vi "SA40144D.20210825 1D+2D.vi"() -> ()   [LabVIEW 2020]
uses:
  <userlib>/LevyLab/XY Utilities/subVIs/Linear Fit (single).vi
  <userlib>/LevyLab/LV to ITX/Data/Data.lvclass
  <userlib>/LevyLab/XY Utilities/xy_utilities.lvlib
panel:
  in  "Tab Control":enum32{"Page 1", "Page 2"}(tab)
  out "G4T vs t  2D":T1(graph)
  out "Temp vs time":T1(graph)
  out "G4T vs t":T1(graph)
  out "G2T vs t":T1(graph)
  out "Arrhenius":cluster{dbl[], dbl[]}[](graph)
  out "E_a":dbl[](array[numeric])
  in  "Source Voltage":dbl=0.1
  in  "Data Folder":path=path "G:/My Drive/ansom/Data/PPMS 2/SA40144D.20210825/45-LockinFieldSweep_hash_16_27_stripe/SA40144D.20210825.000000.dat"
  in  "Trimming":i32=400
  in  "Update":bool
  in  "OK":bool
  out "error out":errorcluster
  in  "error in (no error)":errorcluster
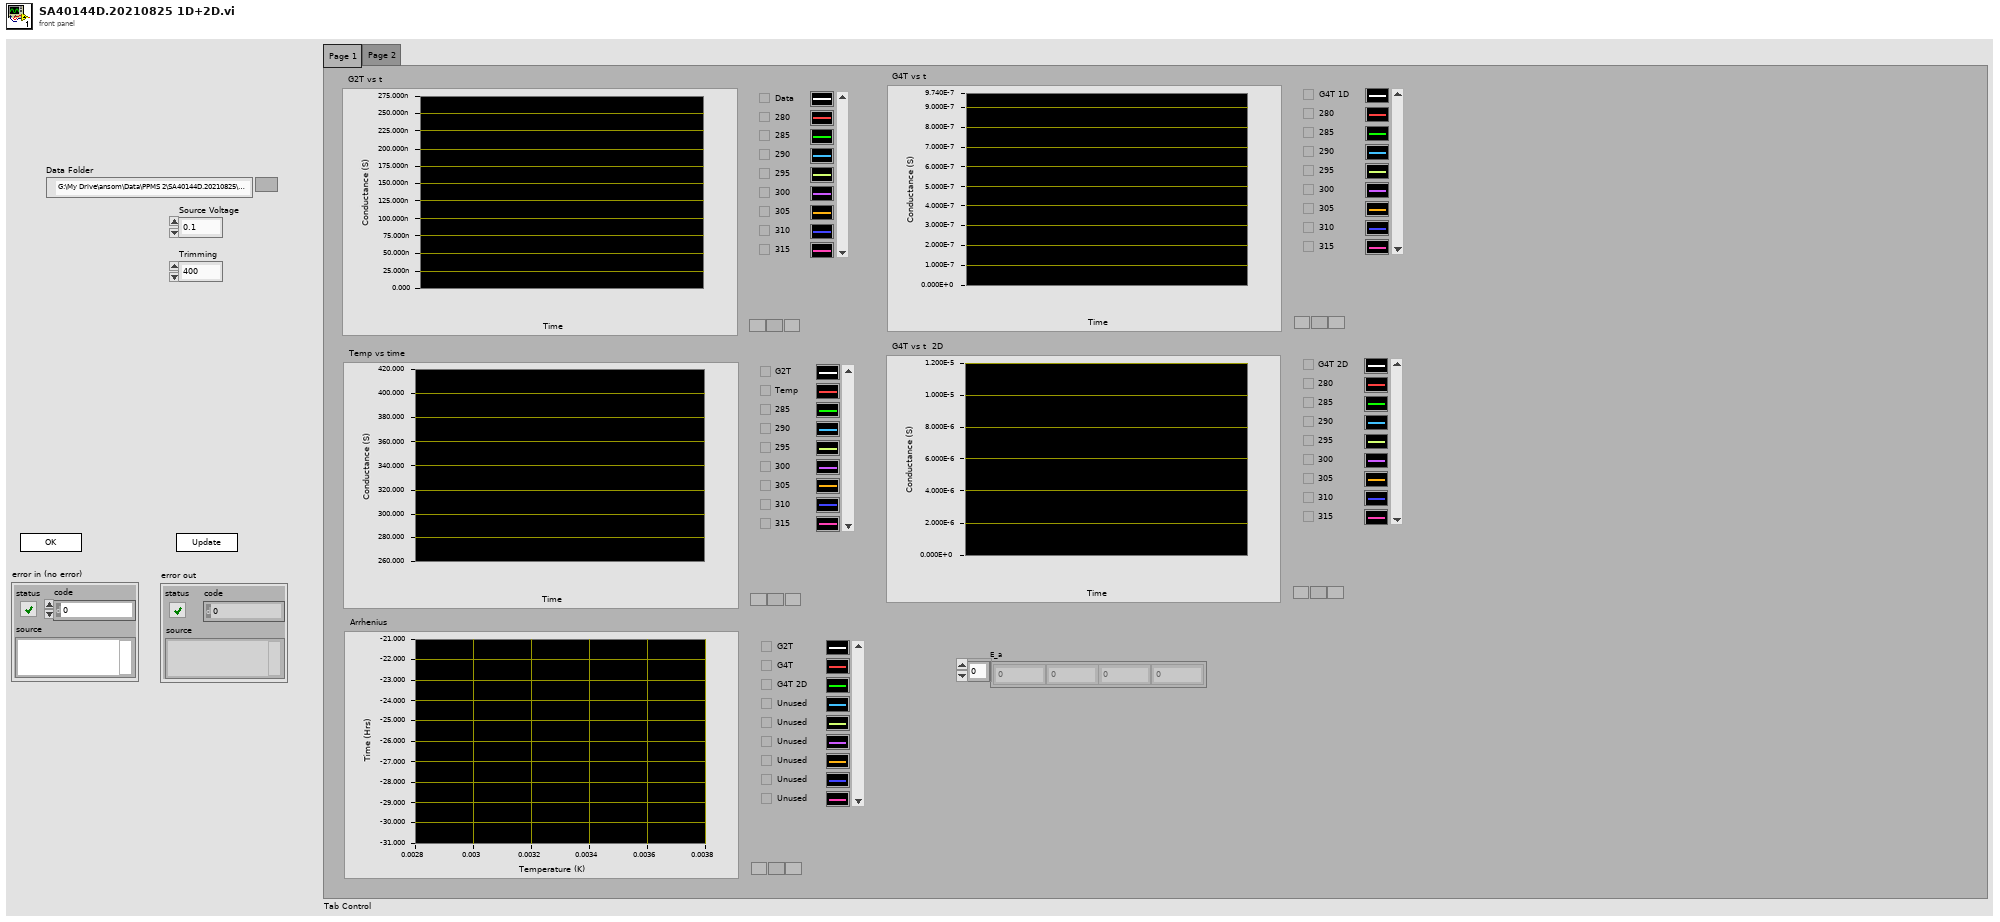
[diagram p1: front panel]
types:
  T1 = cluster{"Data":dbl[], "Best Exponential Fit":dbl[]}[]
  T2 = enum32{"Invalid", "Standard", "Closed", "Hidden", "Minimized", "Maximized"}
  T3 = enum32{"invalid app kind", "Development System", "Run Time System", "Student Edition", "Embedded LabVIEW", "Evaluation", "Custom"}
  T4 = cluster{"Core":cluster{"Current VI Reference":refnum<vi>, "Close Panel on Exit?":bool}, "G2T 1D":cluster{dbl[], dbl[]}[], "G4T 1D":cluster{dbl[], dbl[]}[], "G2T 2D":cluster{dbl[], dbl[]}[], "G4T 2D":cluster{dbl[], dbl[]}[], "Arrhenius":cluster{dbl[], dbl[]}[], "Source Voltage":dbl, "Data Folder":path, "Trimming":i32}
  T5 = cluster{"Current VI Reference":refnum<vi>, "Close Panel on Exit?":bool}
  T6 = typedef "Data.lvclass/Dictionary--cluster.ctl" = cluster{"key":string, "value":variant}
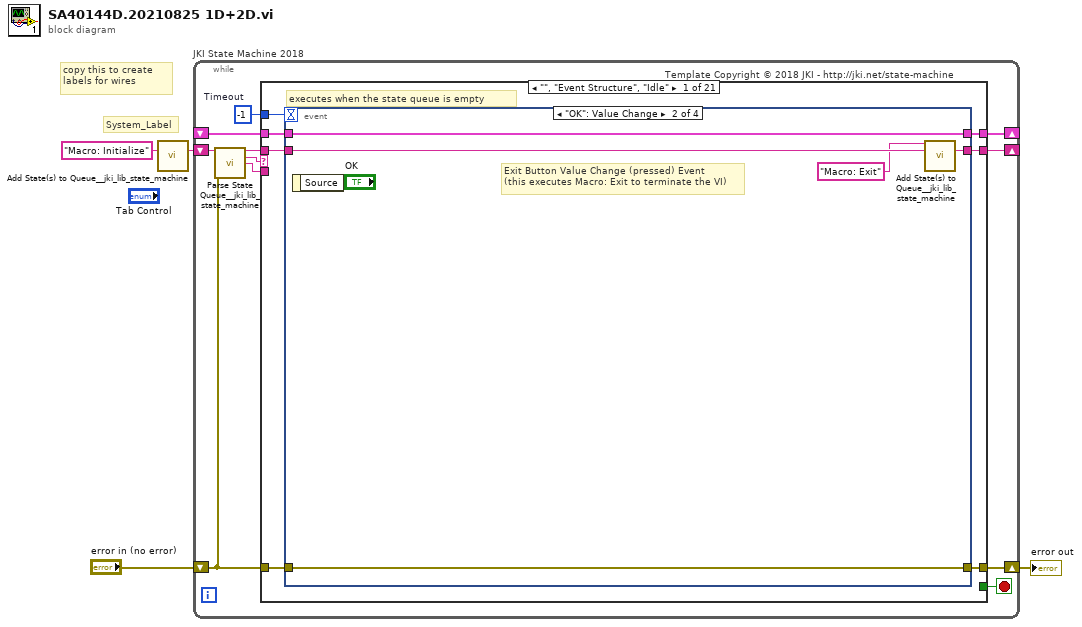
[diagram p0: block diagram]
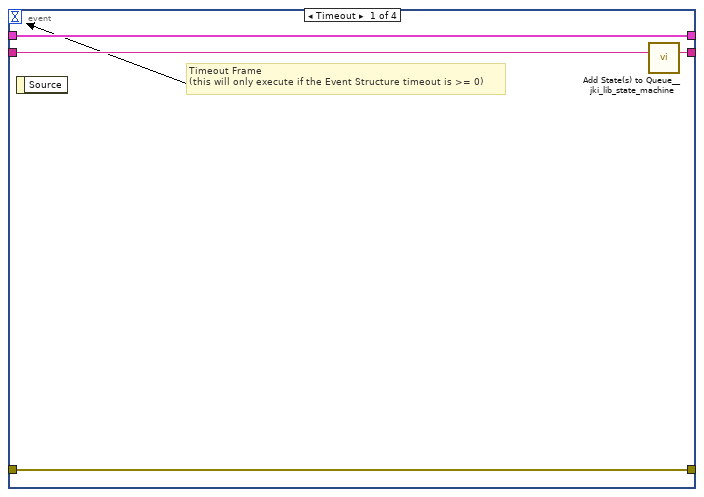
[diagram p2: hidden frame]
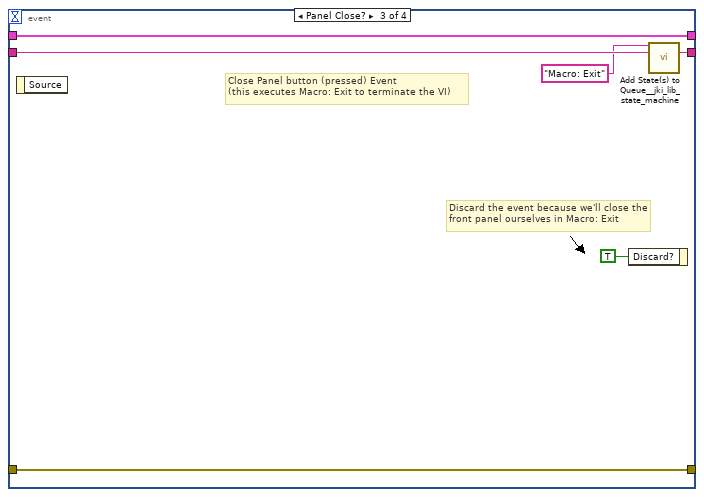
[diagram p3: hidden frame]
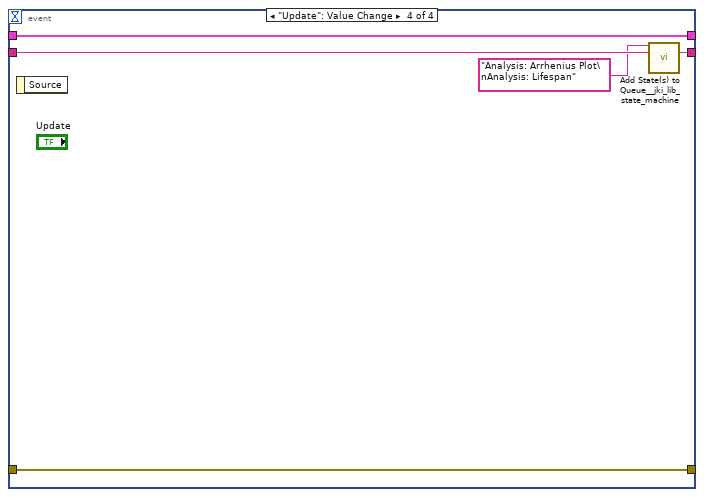
[diagram p4: hidden frame]
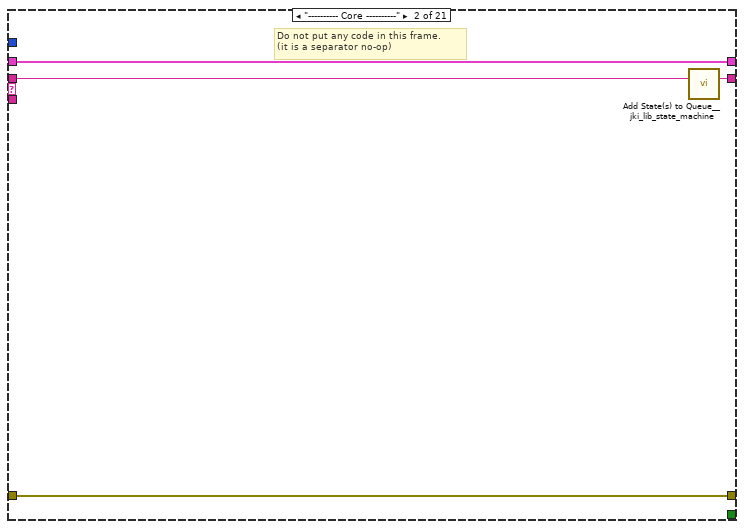
[diagram p5: hidden frame]
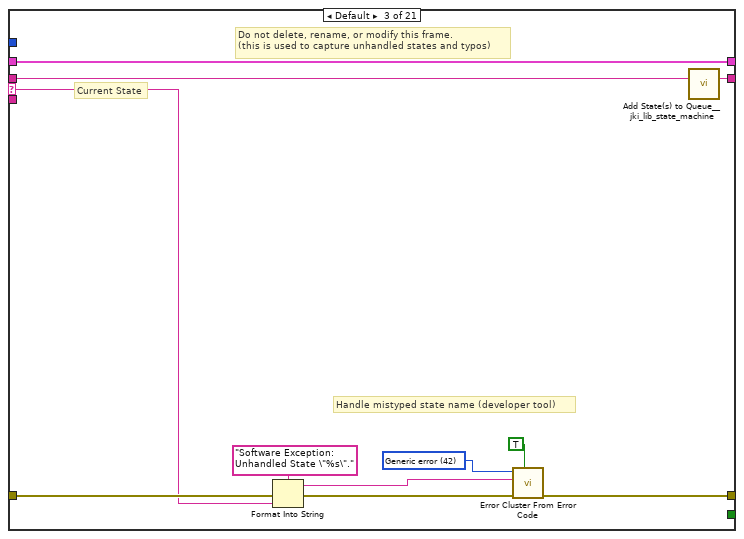
[diagram p6: hidden frame]
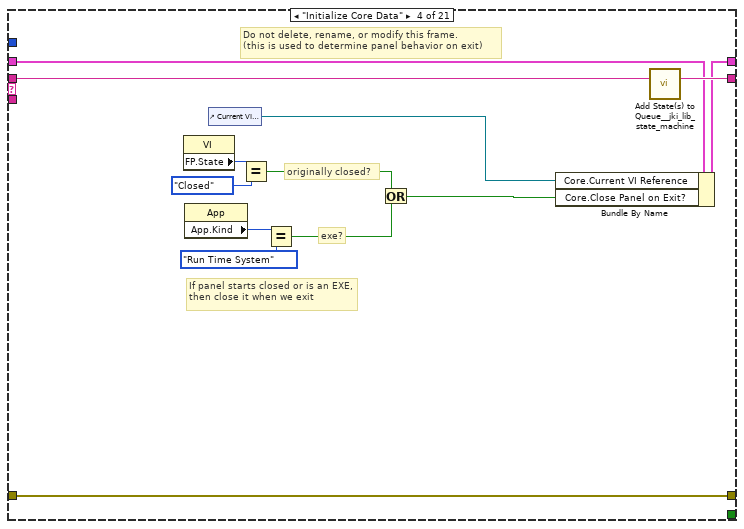
[diagram p7: hidden frame]
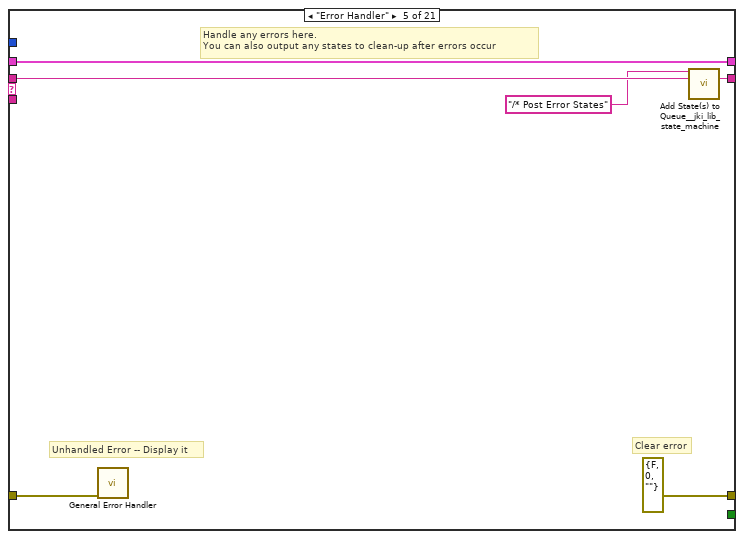
[diagram p8: hidden frame]
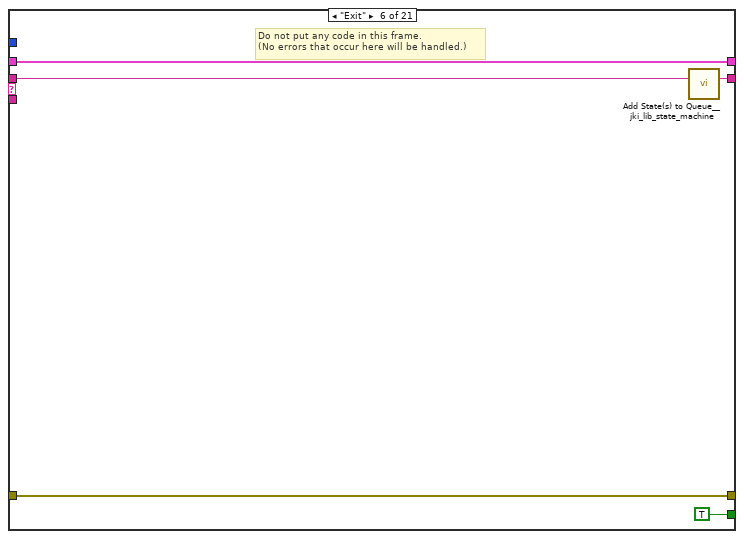
[diagram p9: hidden frame]
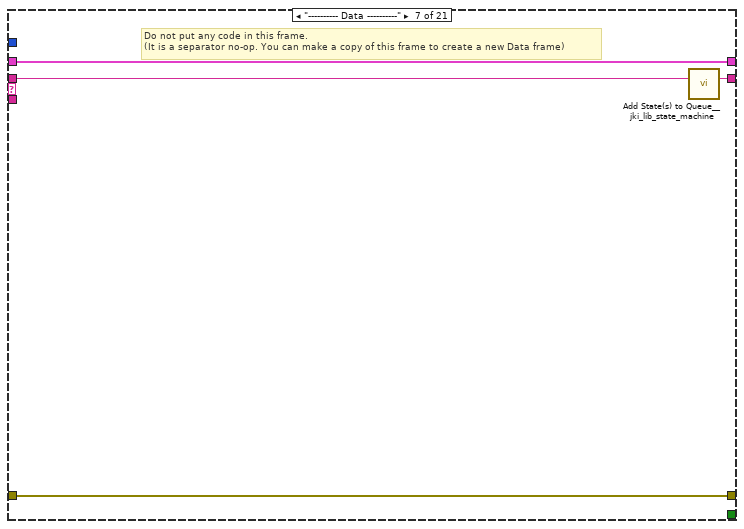
[diagram p10: hidden frame]
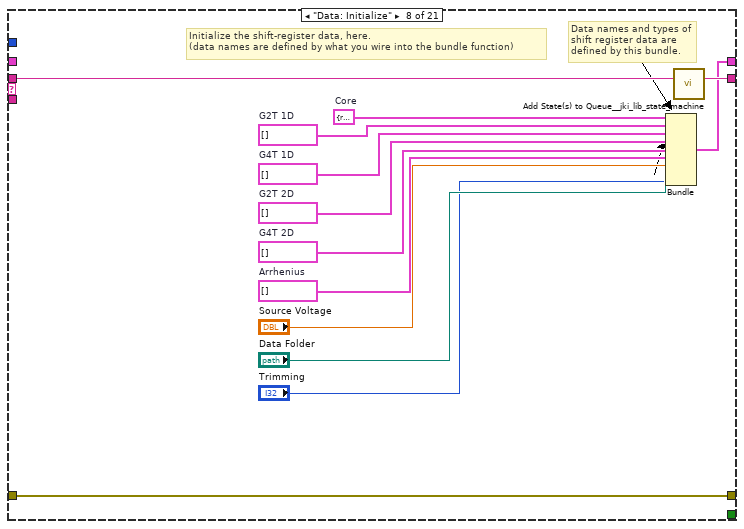
[diagram p11: hidden frame]
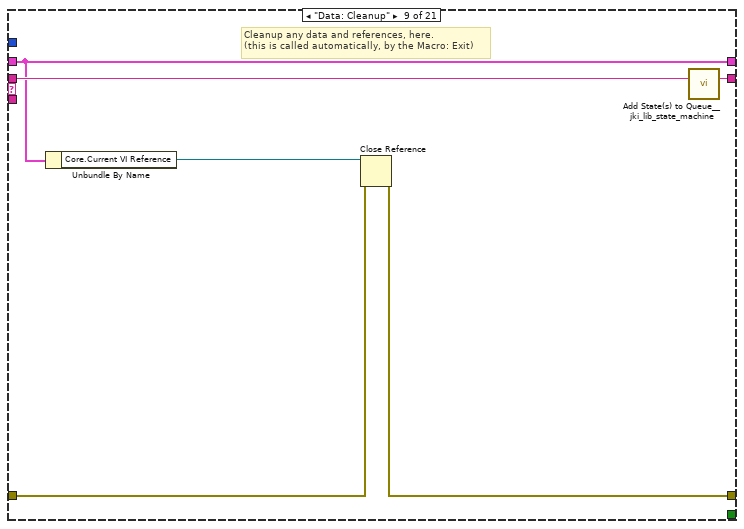
[diagram p12: hidden frame]
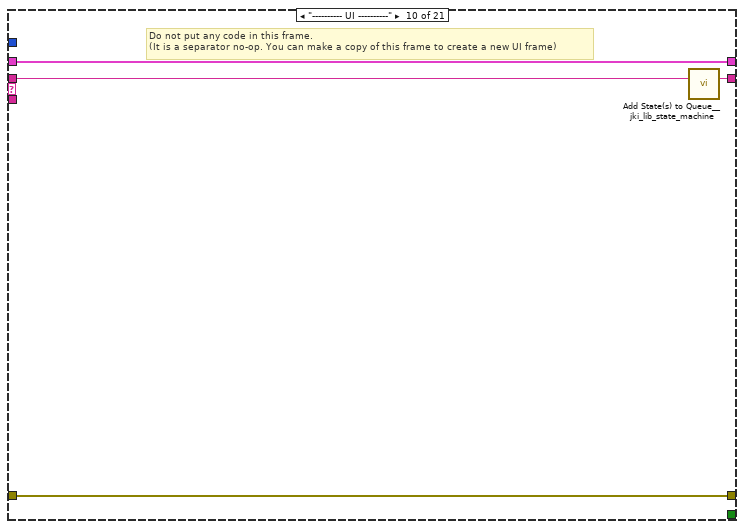
[diagram p13: hidden frame]
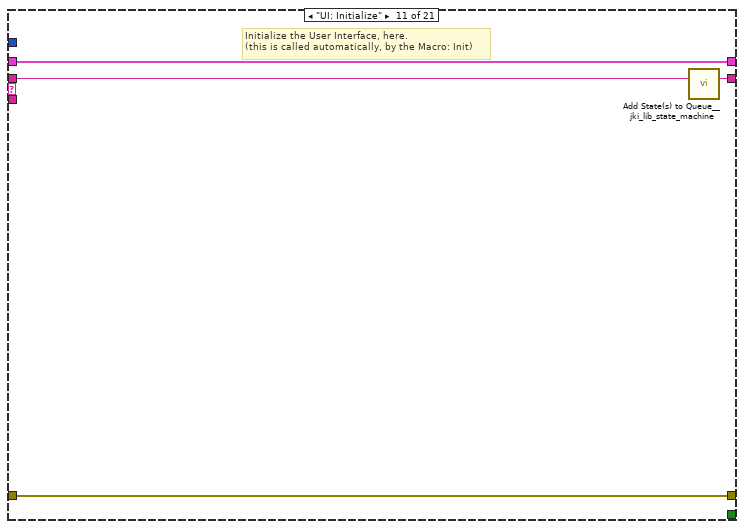
[diagram p14: hidden frame]
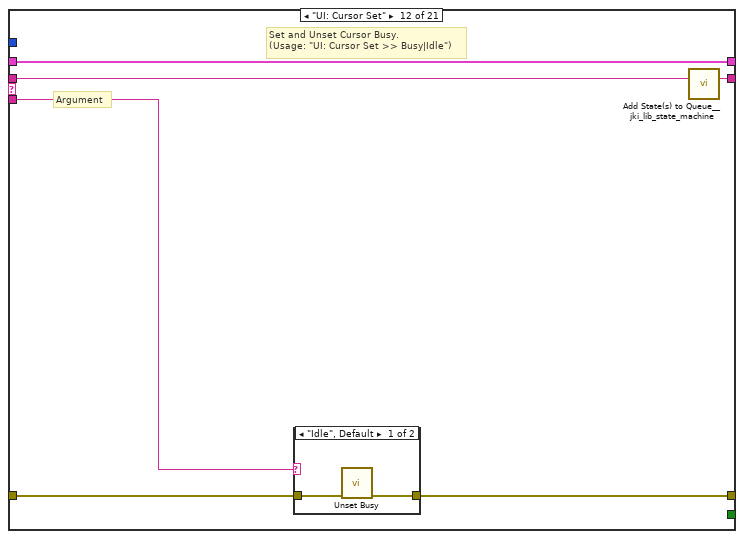
[diagram p15: hidden frame]
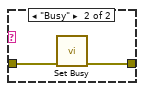
[diagram p16: hidden frame]
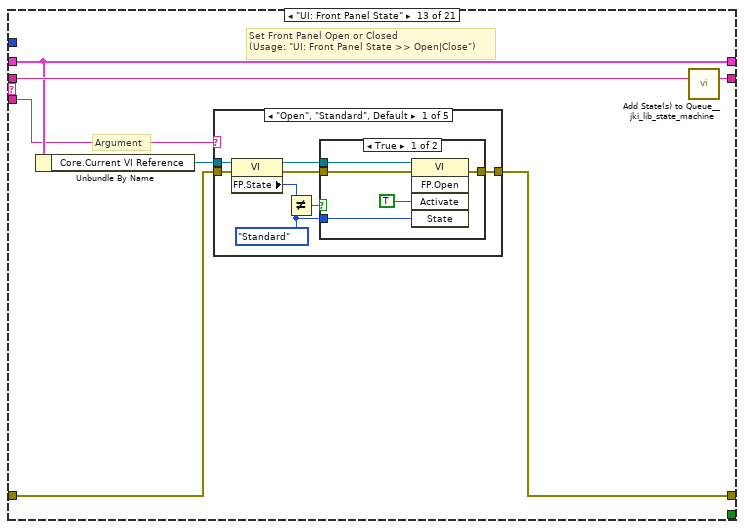
[diagram p17: hidden frame]
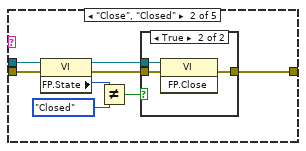
[diagram p19: hidden frame]
diagram:
  # "copy this to create labels for wires"
  # "System_Label"
  n1 = call <vilib>:"Add State(s) to Queue__jki_lib_state_machine.vi"("State(s) in (\"\")"="Macro: Initialize") -> ("States Out"=w4:string)  [unwired: 14 in]
  n2 = while "JKI State Machine 2018" {
    shift-right: [w8] -> _
    shift-left: _ -> [w7]
    shift-right: [w11] -> w1
    shift-left: "error in (no error)" -> [w5]
    shift-right: [w10] -> _
    shift-left: w4 -> [w12]
    stop <- w9 stop-if-true
    w6 = -1  # Timeout
    # "Template Copyright © 2018 JKI - http://jki.net/state-machine"
    n3 = call <vilib>:"Parse State Queue__jki_lib_state_machine.vi"("State Queue"=w12, "Error In (no error)"=w5) -> ("Remaining States"=w14:string, "Current State"=w15:string, "Arguments"=w13:string)  [unwired: 11 in]
    n4 = case shown="\"\", \"Event Structure\", \"Idle\"" w15 {
      selector: w15 -> [_ _ w47 _ _ _ _ _ _ _ _ _ _ _ _ _ _ _ _ _ _]
      tunnel: w14 -> [w22 w46 w51 w70 w76 w81 w85 w98 w104 w108 w112 w118 w129 w198 w203 w213 w217 w249 w280 w292 w311]
      tunnel: w13 -> [_ _ _ _ _ _ _ _ _ _ _ w113 w123 _ _ _ _ _ _ _ _]
      tunnel: w7 -> [w20 w43 w49 w63 w73 w79 w82 _ w99 w105 w110 w116 w125 w195 w200 w210 w214 w245 w276 w289 w296]
      tunnel: [w19 w44 w53 w67 errorcluster {"status"=FALSE, "code"=0, "source"=""} ("error out") w78 w83 w95 w100 w106 w109 w114 w126 w196 w201 w211 w215 w247 w278 w290 w309] -> w11
      tunnel: w5 -> [w18 w44 w52 w67 w72 w78 w83 w95 w101 w106 w109 w115 w127 w196 w201 w211 w215 w247 w278 w290 w309]
      tunnel: [w21 w45 w50 w69 w75 w80 w84 w97 w103 w107 w111 w117 w128 w197 w202 w212 w216 w248 w279 w291 w310] -> w10
      tunnel: [_ _ _ _ _ TRUE _ _ _ _ _ _ _ _ _ _ _ _ _ _ _] -> w9
      tunnel: [w17 w43 w49 w68 w73 w79 w82 w96 w99 w105 w110 w116 w125 w195 w200 w210 w214 w246 w277 w289 w297] -> w8
      tunnel: w6 -> [w16 _ _ _ _ _ _ _ _ _ _ _ _ _ _ _ _ _ _ _ _]
      frame "", "Event Structure", "Idle" {
        # "executes when the state queue is empty"
        n5 = event shown="[1] \"OK\": Value Change" {
          selector: _ -> [_ _ _ _]
          dyn-events: _ -> [_ _ _ _]
          timeout: w16 -> [_ _ _ _]
          tunnel: w22 -> [w26 w31 w37 w41]
          tunnel: [w25 w30 w36 w40] -> w21
          tunnel: w20 -> [w23 w28 w34 w42]
          tunnel: [w24 w29 w35 w38] -> w19
          tunnel: w18 -> [w24 w29 w35 w38]
          tunnel: [w23 w28 w34 w42] -> w17
          event Timeout {
            # "Timeout Frame\n(this will only execute if the Event Structure timeout is >= 0)"
            n6 = event-data() -> ()  [unwired: 1 in, 1 out]
            n7 = call <vilib>:"Add State(s) to Queue__jki_lib_state_machine.vi"("State(s) in (\"\")"=w26) -> ("States Out"=w25:string)  [unwired: 14 in]
          }
          event "OK": Value Change {
            # "Exit Button Value Change (pressed) Event\n(this executes Macro: Exit to terminate the VI)"
            n8 = event-data() -> ()  [unwired: 1 in, 1 out]
            n9 = call <vilib>:"Add State(s) to Queue__jki_lib_state_machine.vi"("State(s) in Front (\"\")"="Macro: Exit", "State(s) in (\"\")"=w31) -> ("States Out"=w30:string)  [unwired: 13 in]
          }
          event Panel Close? {
            # "Discard the event because we'll close the front panel ourselves in Macro: Exit"
            # "Close Panel button (pressed) Event\n(this executes Macro: Exit to terminate the VI)"
            n10 = event-data() -> ()  [unwired: 1 in, 1 out]
            n11 = event-data("Discard?"=TRUE) -> ()  [unwired: 1 in, 1 out]
            n12 = call <vilib>:"Add State(s) to Queue__jki_lib_state_machine.vi"("State(s) in Front (\"\")"="Macro: Exit", "State(s) in (\"\")"=w37) -> ("States Out"=w36:string)  [unwired: 13 in]
          }
          event "Update": Value Change {
            n13 = event-data() -> ()  [unwired: 1 in, 1 out]
            n14 = call <vilib>:"Add State(s) to Queue__jki_lib_state_machine.vi"("State(s) in Front (\"\")"="Analysis: Arrhenius Plot\nAnalysis: Lifespan" ("State(s) in Front (\"\")"), "State(s) in (\"\")"=w41) -> ("States Out"=w40:string)  [unwired: 13 in]
          }
        }
      }
      frame "---------- Core ----------" {
        # "Do not put any code in this frame.\n(it is a separator no-op)"
        n15 = call <vilib>:"Add State(s) to Queue__jki_lib_state_machine.vi"("State(s) in (\"\")"=w46) -> ("States Out"=w45:string)  [unwired: 14 in]
      }
      frame Default {
        w56 = 42 items=["No error", "Argument error", "Memory is full", "Out of zone", "End of file", "File already open", "Generic file I/O error", "File not found", "File permission error", "Disk is full", "Duplicate path", "Too many files open", "System feature not enabled", "Resource file not found", "Cannot add resource", "Resource not found", "Image not found", "Image memory error", "Pen does not exist", "Config type invalid", "Config token not found", "Config parse error", "Config memory error", "Bad external code format", "Bad external code offset", "External code not present", "Null window", "Destroy window error", "Null menu", "Print aborted", "Bad print record", "Print driver error", "Windows error during printing", "Memory error during printing", "Print dialog error", "Generic print error", "Invalid device refnum", "Device not found", "Device parameter error", "Device unit error", "Cannot open device", "Device call aborted", "Generic error", "Cancelled by user", "Object ID too low", "Object ID too high", "Object not in heap", "Unknown heap", "Unknown object (invalid DefProc)", "Unknown object (DefProc not in table)", "Message out of range", "Invalid (null) method", "Unknown message", "Manager call not supported", "Bad address", "Network operation in progress", "Network operation timed out", "Connection is busy", "Network attribute not supported", "Network error", "Address in use", "System out of memory", "Connection aborted", "Connection refused", "Not connected", "Already connected", "Connection closed", "Initialization error (interapplication manager)", "Bad occurrence", "Wait on unbound occurrence handler", "Occurrence queue overflow", "Datalog type conflict", "Unused", "Unrecognized type (interapplication manager)", "Memory corrupt", "Failed to make temporary DLL", "Old CIN version", "Drag socket not found", "Failed to load drop-object", "Failed to register OLE object", "Failed to release OLE object", "Format specifier type mismatch", "Unknown format specifier", "Too few format specifiers", "Too many format specifiers", "Scan failed", "Newer CIN version", "Error converting to variant", "Runtime menu error", "Password tampered", "Variant attribute not found", "Incompatible variant data type", "Event data is not available", "Event Store is not present", "Occurrence is not found", "Event Queue is not created", "Event info is not available", "Refnum passed is NULL", "Error retrieving Class GUID", "Error retrieving CoClass GUID", "Error retrieving TypeLib GUID.", "Bad built application magic bytes.", "Specific driver is different from the specific driver associated with the Logical Name.", "There is no session opened to the class driver.", "Max Error", "MAX - Error with config objects", "MAX - Error loading configuration", "MAX - Group not supported"]
        # "Current State"
        # "Do not delete, rename, or modify this frame.\n(this is used to capture unhandled states and typos)"
        # "Handle mistyped state name (developer tool)"
        n16 = Format Into String(format string="Software Exception: Unhandled State \"%s\"." ("message"), error in=w52, w47) -> (resulting string=w55:string, error out=w54:errorcluster)  [unwired: 1 in]
        n17 = call <vilib>:"Error Cluster From Error Code.vi"("show call chain? (False)"=TRUE, "error in (no error)"=w54, "error message (\"\")"=w55, "error code (0)"=w56) -> ("error out"=w53:errorcluster)  [unwired: 5 in]
        n18 = call <vilib>:"Add State(s) to Queue__jki_lib_state_machine.vi"("State(s) in (\"\")"=w51) -> ("States Out"=w50:string)  [unwired: 14 in]
      }
      frame "Initialize Core Data" {
        # "Do not delete, rename, or modify this frame.\n(this is used to determine panel behavior on exit)"
        # "originally closed?"
        # "exe?"
        # "If panel starts closed or is an EXE, then close it when we exit"
        n19 = property class="VI"() -> ("FP.State"=w60:T2)  [unwired: 2 in, 2 out]
        n20 = property class="App"() -> ("App.Kind"=w66:T3)  [unwired: 2 in, 2 out]
        n21 = control-ref of="Current VI Reference"() -> (w61:refnum<vi>)
        n22 = Equal?(x=w60, y=T2."Closed" ("Front Panel Window:State")) -> (x = y?=w58:bool)
        n23 = Equal?(x=w66, y=T3."Run Time System" ("Application:Kind")) -> (x = y?=w64:bool)
        n24 = Or(x=w58, y=w64) -> (x .or. y?=w62:bool)
        n25 = Bundle By Name(cluster=w63, "Core.Current VI Reference"=w61, "Core.Close Panel on Exit?"=w62) -> (w68:T4)
        n26 = call <vilib>:"Add State(s) to Queue__jki_lib_state_machine.vi"("State(s) in (\"\")"=w70) -> ("States Out"=w69:string)  [unwired: 14 in]
      }
      frame "Error Handler" {
        # "Unhandled Error -- Display it"
        # "Handle any errors here.\nYou can also output any states to clean-up after errors occur"
        # "Clear error"
        n27 = call <vilib>:"General Error Handler.vi"("error in (no error)"=w72) -> ()  [unwired: 10 in, 5 out]
        n28 = call <vilib>:"Add State(s) to Queue__jki_lib_state_machine.vi"("State(s) in Front (\"\")"="/* Post Error States", "State(s) in (\"\")"=w76) -> ("States Out"=w75:string)  [unwired: 13 in]
      }
      frame "Exit" {
        # "Do not put any code in this frame.\n(No errors that occur here will be handled.)"
        n29 = call <vilib>:"Add State(s) to Queue__jki_lib_state_machine.vi"("State(s) in (\"\")"=w81) -> ("States Out"=w80:string)  [unwired: 14 in]
      }
      frame "---------- Data ----------" {
        # "Do not put any code in this frame.\n(It is a separator no-op. You can make a copy of this frame to create a new Data frame)"
        n30 = call <vilib>:"Add State(s) to Queue__jki_lib_state_machine.vi"("State(s) in (\"\")"=w85) -> ("States Out"=w84:string)  [unwired: 14 in]
      }
      frame "Data: Initialize" {
        w86 = cluster{dbl[], dbl[]}[] []  # Arrhenius
        w92 = cluster{dbl[], dbl[]}[] []  # G4T 2D
        w91 = cluster{dbl[], dbl[]}[] []  # G2T 2D
        w90 = cluster{dbl[], dbl[]}[] []  # G4T 1D
        w89 = cluster{dbl[], dbl[]}[] []  # G2T 1D
        w94 = T5 {"Current VI Reference"=refnum, "Close Panel on Exit?"=FALSE}  # Core
        # "Data names and types of shift register data are defined by this bundle."
        # "Initialize the shift-register data, here.\n(data names are defined by what you wire into the bundle function)"
        n31 = Bundle("Core"=w94, "G2T 1D"=w89, "G4T 1D"=w90, "G2T 2D"=w91, "G4T 2D"=w92, "Arrhenius"=w86, "Source Voltage"="Source Voltage", "Data Folder"="Data Folder", "Trimming"="Trimming") -> (w96:T4)  [unwired: 1 in]
        n32 = call <vilib>:"Add State(s) to Queue__jki_lib_state_machine.vi"("State(s) in (\"\")"=w98) -> ("States Out"=w97:string)  [unwired: 14 in]
      }
      frame "Data: Cleanup" {
        # "Cleanup any data and references, here.\n(this is called automatically, by the Macro: Exit)"
        n33 = Unbundle By Name(w99) -> ("Core.Current VI Reference"=w102:refnum<vi>)
        n34 = Close Reference(reference=w102, error in (no error)=w101) -> (error out=w100:errorcluster)
        n35 = call <vilib>:"Add State(s) to Queue__jki_lib_state_machine.vi"("State(s) in (\"\")"=w104) -> ("States Out"=w103:string)  [unwired: 14 in]
      }
      frame "---------- UI ----------" {
        # "Do not put any code in this frame.\n(It is a separator no-op. You can make a copy of this frame to create a new UI frame)"
        n36 = call <vilib>:"Add State(s) to Queue__jki_lib_state_machine.vi"("State(s) in (\"\")"=w108) -> ("States Out"=w107:string)  [unwired: 14 in]
      }
      frame "UI: Initialize" {
        # "Initialize the User Interface, here.\n(this is called automatically, by the Macro: Init)"
        n37 = call <vilib>:"Add State(s) to Queue__jki_lib_state_machine.vi"("State(s) in (\"\")"=w112) -> ("States Out"=w111:string)  [unwired: 14 in]
      }
      frame "UI: Cursor Set" {
        # "Argument"
        # "Set and Unset Cursor Busy.\n(Usage: \"UI: Cursor Set >> Busy|Idle\")"
        n38 = case shown="\"Idle\", Default" w113 {
          tunnel: w115 -> [w120 w122]
          tunnel: [w119 w121] -> w114
          frame "Idle", Default {
            n39 = call <vilib>:"Unset Busy.vi"("error in (no error)"=w120) -> ("error out"=w119:errorcluster)  [unwired: 10 in]
          }
          frame "Busy" {
            n40 = call <vilib>:"Set Busy.vi"("error in (no error)"=w122) -> ("error out"=w121:errorcluster)  [unwired: 9 in, 1 out]
          }
        }
        n41 = call <vilib>:"Add State(s) to Queue__jki_lib_state_machine.vi"("State(s) in (\"\")"=w118) -> ("States Out"=w117:string)  [unwired: 14 in]
      }
      frame "UI: Front Panel State" {
        # "Argument"
        # "Set Front Panel Open or Closed\n(Usage: \"UI: Front Panel State >> Open|Close\")"
        n42 = Unbundle By Name(w125) -> ("Core.Current VI Reference"=w124:refnum<vi>)
        n43 = case shown="\"Open\", \"Standard\", Default" w123 {
          tunnel: w127 -> [w135 w150 w161 w174 w187]
          tunnel: [w137 w151 w163 w176 w189] -> w126
          tunnel: w124 -> [w136 w148 w162 w175 w188]
          frame "Open", "Standard", Default {
            w130 = T2."Standard" ("State")
            n44 = property class="VI"(reference=w136, error in=w135) -> (reference out=w133:refnum<vi>, error out=w134:errorcluster, "FP.State"=w132:T2)
            n45 = Not Equal?(x=w132, y=w130) -> (x != y?=w131:bool)
            n46 = case shown="True" w131 {
              tunnel: [w141 w143] -> w137
              tunnel: w134 -> [w140 w143]
              tunnel: w133 -> [w139 _]
              tunnel: w130 -> [w138 _]
              frame True {
                n47 = invoke class="VI" method="FP.Open"(reference=w139, error in=w140, "Activate"=TRUE, "State"=w138) -> (error out=w141:errorcluster)  [unwired: 1 in, 4 out]
              }
              frame False {
              }
            }
          }
          frame "Close", "Closed" {
            n48 = property class="VI"(reference=w148, error in=w150) -> (reference out=w147:refnum<vi>, error out=w149:errorcluster, "FP.State"=w145:T2)
            n49 = Not Equal?(x=w145, y=T2."Closed" ("Front Panel Window:State")) -> (x != y?=w144:bool)
            n50 = case shown="True" w144 {
              tunnel: [w152 w155] -> w151
              tunnel: w149 -> [w152 w154]
              tunnel: w147 -> [_ w153]
              frame False {
              }
              frame True {
                n51 = invoke class="VI" method="FP.Close"(reference=w153, error in=w154) -> (error out=w155:errorcluster)  [unwired: 1 in, 2 out]
              }
            }
          }
          frame "Hidden", "Hide" {
            w156 = T2."Hidden" ("State")
            n52 = property class="VI"(reference=w162, error in=w161) -> (reference out=w159:refnum<vi>, error out=w160:errorcluster, "FP.State"=w158:T2)
            n53 = Not Equal?(x=w158, y=w156) -> (x != y?=w157:bool)
            n54 = case shown="True" w157 {
              tunnel: [w167 w168] -> w163
              tunnel: w160 -> [w166 w168]
              tunnel: w159 -> [w165 _]
              tunnel: w156 -> [w164 _]
              frame True {
                n55 = invoke class="VI" method="FP.Open"(reference=w165, error in=w166, "State"=w164) -> (error out=w167:errorcluster)  [unwired: 2 in, 4 out]
              }
              frame False {
              }
            }
          }
          frame "Minimize", "Minimized" {
            w169 = T2."Minimized" ("State")
            n56 = property class="VI"(reference=w175, error in=w174) -> (reference out=w172:refnum<vi>, error out=w173:errorcluster, "FP.State"=w171:T2)
            n57 = Not Equal?(x=w171, y=w169) -> (x != y?=w170:bool)
            n58 = case shown="True" w170 {
              tunnel: [w180 w181] -> w176
              tunnel: w173 -> [w179 w181]
              tunnel: w172 -> [w178 _]
              tunnel: w169 -> [w177 _]
              frame True {
                n59 = invoke class="VI" method="FP.Open"(reference=w178, error in=w179, "State"=w177) -> (error out=w180:errorcluster)  [unwired: 2 in, 4 out]
              }
              frame False {
              }
            }
          }
          frame "Maximize", "Maximized" {
            w182 = T2."Maximized" ("State")
            n60 = property class="VI"(reference=w188, error in=w187) -> (reference out=w185:refnum<vi>, error out=w186:errorcluster, "FP.State"=w184:T2)
            n61 = Not Equal?(x=w184, y=w182) -> (x != y?=w183:bool)
            n62 = case shown="True" w183 {
              tunnel: [w193 w194] -> w189
              tunnel: w186 -> [w192 w194]
              tunnel: w185 -> [w191 _]
              tunnel: w182 -> [w190 _]
              frame True {
                n63 = invoke class="VI" method="FP.Open"(reference=w191, error in=w192, "State"=w190) -> (error out=w193:errorcluster)  [unwired: 2 in, 4 out]
              }
              frame False {
              }
            }
          }
        }
        n64 = call <vilib>:"Add State(s) to Queue__jki_lib_state_machine.vi"("State(s) in (\"\")"=w129) -> ("States Out"=w128:string)  [unwired: 14 in]
      }
      frame "---------- Macro ----------" {
        # "Do not put any code in this frame.\n(It is a separator no-op. You can make a copy of this frame to create a new Macro frame)"
        n65 = call <vilib>:"Add State(s) to Queue__jki_lib_state_machine.vi"("State(s) in (\"\")"=w198) -> ("States Out"=w197:string)  [unwired: 14 in]
      }
      frame "Macro: Initialize" {
        # "Initialization Macro\n(This is called once, when the VI starts)"
        n66 = call <vilib>:"Add State(s) to Queue__jki_lib_state_machine.vi"("State(s) in Front (\"\")"="Data: Initialize\nInitialize Core Data\nUI: Initialize\nUI: Front Panel State >> Open\nAnalysis: Load 1D\nAnalysis: Load 2D\nAnalysis: Arrhenius (no BG)\nAnalysis: Plot G vs t\n\n# Analysis: Lifespan", "State(s) in (\"\")"=w203) -> ("States Out"=w202:string)  [unwired: 13 in]
      }
      frame "Macro: Exit" {
        # "Exit Macro\n(This is called once, when the VI exits)"
        n67 = Unbundle By Name(w210) -> ("Core.Close Panel on Exit?"=w209:bool)
        n68 = Select(t="UI: Front Panel State >> Close", s=w209, f="") -> (s? t:f=w206:string)
        n69 = call <vilib>:"Add State(s) to Queue__jki_lib_state_machine.vi"("State(s) in (\"\")"=w206, "State(s) at Back (\"\")"="Data: Cleanup\nExit") -> ("States Out"=w204:string)  [unwired: 13 in]
        n70 = call <vilib>:"Add State(s) to Queue__jki_lib_state_machine.vi"("State(s) in Front (\"\")"=w204, "State(s) in (\"\")"=w213) -> ("States Out"=w212:string)  [unwired: 13 in]
      }
      frame "---------- Analysis ----------" {
        # "Template Separator\n(You can make a copy of, or modify, this frame)"
        n71 = call <vilib>:"Add State(s) to Queue__jki_lib_state_machine.vi"("State(s) in (\"\")"=w217) -> ("States Out"=w216:string)  [unwired: 14 in]
      }
      frame "Analysis: Load 1D" {
        # "G2T = X3/V_s\nG4T = X3/(X5-X4)"
        n72 = Unbundle By Name(w245) -> ("Source Voltage"=w225:dbl, "Data Folder"=w219:path)
        n73 = call <userlib>:"Data Read.vi"("path"=w219) -> ("Data (Dictionary)"=w243:T6[])  [unwired: 7 in, 3 out]
        n74 = call "Read Dictionary.vi"("Numeric"=0, "Dictionary In"=w243) -> ("data"=w239:dbl[])
        n75 = call "Read Dictionary.vi"("Numeric"=5, "Dictionary In"=w243) -> ("data"=w233:dbl[])
        n76 = call "Read Dictionary.vi"("Numeric"=7 ("index"), "Dictionary In"=w243) -> ("data"=w234:dbl[])
        n77 = call "Read Dictionary.vi"("Numeric"=6, "Dictionary In"=w243) -> ("data"=w238:dbl[])
        n78 = call "Read Dictionary.vi"("Numeric"=1, "Dictionary In"=w243) -> ("data"=w237:dbl[])
        n79 = Array Subset(array=w239) -> (w232:dbl[])  [unwired: 2 in]
        n80 = Array Subset(array=w233) -> (w228:dbl[])  [unwired: 2 in]
        n81 = Array Subset(array=w234) -> (w230:dbl[])  [unwired: 2 in]
        n82 = Array Subset(array=w238) -> (w229:dbl[])  [unwired: 2 in]
        n83 = Subtract(x=w230, y=w229) -> (x-y=w227:dbl[])
        n84 = Divide(x=w228, y=w225) -> (x/y=w231:dbl[])
        n85 = Divide(x=w228, y=w227) -> (x/y=w226:dbl[])
        n86 = Array Subset(array=w237) -> (w244:dbl[])  [unwired: 2 in]
        n87 = Absolute Value(x=w226) -> (abs(x)=w218:dbl[])
        n88 = Bundle(w232, w231) -> (w223:cluster{dbl[], dbl[]})  [unwired: 1 in]
        n89 = Bundle(w232, w244) -> (w220:cluster{dbl[], dbl[]})  [unwired: 1 in]
        n90 = Bundle(w232, w218) -> (w224:cluster{dbl[], dbl[]})  [unwired: 1 in]
        n91 = Build Array(w223, w220) -> (w222:cluster{dbl[], dbl[]}[])
        n92 = Build Array(w224, w220) -> (w221:cluster{dbl[], dbl[]}[])
        n93 = call <vilib>:"Add State(s) to Queue__jki_lib_state_machine.vi"("State(s) in (\"\")"=w249) -> ("States Out"=w248:string)  [unwired: 14 in]
        n94 = Bundle By Name(cluster=w245, "G2T 1D"=w222, "G4T 1D"=w221) -> (w246:T4)
      }
      frame "Analysis: Load 2D" {
        # "G2T = X3/V_s\nG4T = X3/(X8-X1)"
        n95 = Unbundle By Name(w276) -> ("Source Voltage"=w261:dbl, "Data Folder"=w250:path)
        n96 = call <userlib>:"Data Read.vi"("path"=w250) -> ("Data (Dictionary)"=w257:T6[])  [unwired: 7 in, 3 out]
        n97 = call "Read Dictionary.vi"("Numeric"=0, "Dictionary In"=w257) -> ("data"=w275:dbl[])
        n98 = call "Read Dictionary.vi"("Numeric"=5, "Dictionary In"=w257) -> ("data"=w272:dbl[])
        n99 = call "Read Dictionary.vi"("Numeric"=3 ("index"), "Dictionary In"=w257) -> ("data"=w273:dbl[])
        n100 = call "Read Dictionary.vi"("Numeric"=4, "Dictionary In"=w257) -> ("data"=w274:dbl[])
        n101 = call "Read Dictionary.vi"("Numeric"=1, "Dictionary In"=w257) -> ("data"=w258:dbl[])
        n102 = Array Subset(array=w275) -> (w256:dbl[])  [unwired: 2 in]
        n103 = Array Subset(array=w272) -> (w266:dbl[])  [unwired: 2 in]
        n104 = Array Subset(array=w273) -> (w265:dbl[])  [unwired: 2 in]
        n105 = Array Subset(array=w274) -> (w264:dbl[])  [unwired: 2 in]
        n106 = Subtract(x=w265, y=w264) -> (x-y=w267:dbl[])
        n107 = Array Subset(array=w258) -> (w260:dbl[])  [unwired: 2 in]
        n108 = Divide(x=w266, y=w261) -> (x/y=w262:dbl[])
        n109 = Divide(x=w266, y=w267) -> (x/y=w263:dbl[])
        n110 = Bundle(w256, w260) -> (w254:cluster{dbl[], dbl[]})  [unwired: 1 in]
        n111 = Bundle(w256, w262) -> (w255:cluster{dbl[], dbl[]})  [unwired: 1 in]
        n112 = Bundle(w256, w263) -> (w253:cluster{dbl[], dbl[]})  [unwired: 1 in]
        n113 = Build Array(w255, w254) -> (w252:cluster{dbl[], dbl[]}[])
        n114 = Build Array(w253, w254) -> (w251:cluster{dbl[], dbl[]}[])
        n115 = call <vilib>:"Add State(s) to Queue__jki_lib_state_machine.vi"("State(s) in (\"\")"=w280) -> ("States Out"=w279:string)  [unwired: 14 in]
        n116 = Bundle By Name(cluster=w276, "G2T 2D"=w252, "G4T 2D"=w251) -> (w277:T4)
      }
      frame "Analysis: Plot G vs t" {
        n117 = Unbundle By Name(w289) -> ("G2T 1D"=→"G2T vs t":cluster{dbl[], dbl[]}[], "G4T 1D"=→"G4T vs t":cluster{dbl[], dbl[]}[], "G2T 2D"=→"Temp vs time":cluster{dbl[], dbl[]}[], "G4T 2D"=→"G4T vs t  2D":cluster{dbl[], dbl[]}[], "Arrhenius"=w284:cluster{dbl[], dbl[]}[])
        "Arrhenius" <- w284
        n118 = for {
          tunnel: w284 -> [w294] mode=indexing
          tunnel: [w293] -> w281 mode=indexing
          n119 = call-poly <userlib>:"Linear Fit.vi"("XY-data"=w294) -> ("slope"=w293:dbl)  [unwired: 4 in, 6 out]
        }
        n120 = Multiply(x=w281, y=8.617333e-05) -> (x*y=→"E_a":dbl[])
        n121 = call <vilib>:"Add State(s) to Queue__jki_lib_state_machine.vi"("State(s) in (\"\")"=w292) -> ("States Out"=w291:string)  [unwired: 14 in]
      }
      frame "Analysis: Arrhenius (no BG)" {
        # "Template Separator\n(You can make a copy of, or modify, this frame)"
        n122 = Unbundle By Name(w296) -> ("G2T 1D"=w308:cluster{dbl[], dbl[]}[], "G4T 1D"=w307:cluster{dbl[], dbl[]}[], "G4T 2D"=w306:cluster{dbl[], dbl[]}[])
        n123 = for {
          tunnel: w308 -> [w344]
          tunnel: w307 -> [w343]
          tunnel: w306 -> [w341]
          tunnel: dbl[] [275.0, 280.0, 285.0, 290.0, 295.0, 300.0, 305.0, 310.0, 315.0, 320.0, 325.0, 330.0, 335.0, 340.0] -> [w313] mode=indexing
          tunnel: [w312] -> w301 mode=indexing
          tunnel: [w322] -> w303 mode=indexing
          tunnel: [w316] -> w302 mode=indexing
          tunnel: [w319] -> w304 mode=indexing
          w336 = dbl[] []
          w342 = 0
          n124 = Index Array(array=w344, index=w342) -> (element=w334:cluster{dbl[], dbl[]})
          n125 = Index Array(array=w343, index=w342) -> (element=w333:cluster{dbl[], dbl[]})
          n126 = Index Array(array=w341, index=w342) -> (element=w335:cluster{dbl[], dbl[]})
          n127 = Index Array(array=w341, index=1) -> (element=w339:cluster{dbl[], dbl[]})
          n128 = Unbundle(w334) -> (w330:dbl[])  [unwired: 1 out]
          n129 = Unbundle(w333) -> (w331:dbl[])  [unwired: 1 out]
          n130 = Unbundle(w335) -> (w332:dbl[])  [unwired: 1 out]
          n131 = Unbundle(w339) -> (w338:dbl[], w337:dbl[])
          n132 = for {
            tunnel: w313 -> [w360]
            tunnel: w337 -> [w359] mode=indexing
            shift-right: [w354] -> w329
            shift-left: w336 -> [w355]
            tunnel: w338 -> [w356] mode=indexing
            shift-right: [w350] -> w326
            shift-left: w336 -> [w351]
            shift-right: [w352] -> w327
            shift-left: w336 -> [w353]
            shift-right: [w348] -> w328
            shift-left: w336 -> [w349]
            tunnel: w332 -> [w347] mode=indexing
            tunnel: w331 -> [w346] mode=indexing
            tunnel: w330 -> [w345] mode=indexing
            n133 = call "In Temp Range"("Within"=0.02, "Target"=w360, "Data"=w359) -> ("In Range?"=w357:bool)
            n134 = case shown="True" w357 {
              tunnel: w356 -> [_ w376]
              tunnel: w355 -> [w364 w375]
              tunnel: [w364 w374] -> w354
              tunnel: w353 -> [w363 w373]
              tunnel: [w363 w372] -> w352
              tunnel: w351 -> [w362 w371]
              tunnel: [w362 w370] -> w350
              tunnel: w349 -> [w361 w369]
              tunnel: [w361 w368] -> w348
              tunnel: w347 -> [_ w367]
              tunnel: w346 -> [_ w366]
              tunnel: w345 -> [_ w365]
              frame False {
              }
              frame True {
                n135 = Insert Into Array(array=w369, new element=w365) -> (w368:dbl[])  [unwired: 1 in]
                n136 = Insert Into Array(array=w371, new element=w366) -> (w370:dbl[])  [unwired: 1 in]
                n137 = Insert Into Array(array=w373, new element=w367) -> (w372:dbl[])  [unwired: 1 in]
                n138 = Insert Into Array(array=w375, new element=w376) -> (w374:dbl[])  [unwired: 1 in]
              }
            }
          }
          n139 = Bundle(w329, w328) -> (w323:cluster{dbl[], dbl[]})  [unwired: 1 in]
          n140 = Bundle(w329, w326) -> (w324:cluster{dbl[], dbl[]})  [unwired: 1 in]
          n141 = Bundle(w329, w327) -> (w325:cluster{dbl[], dbl[]})  [unwired: 1 in]
          n142 = Reciprocal(x=w313) -> (1/x=w312:dbl)
          n143 = call-poly <userlib>:"Linear Fit.vi"("XY-data"=w323) -> ("slope"=w317:dbl)  [unwired: 4 in, 6 out]
          n144 = call-poly <userlib>:"Linear Fit.vi"("XY-data"=w324) -> ("slope"=w314:dbl)  [unwired: 4 in, 6 out]
          n145 = call-poly <userlib>:"Linear Fit.vi"("XY-data"=w325) -> ("slope"=w320:dbl)  [unwired: 4 in, 6 out]
          n146 = Absolute Value(x=w314) -> (abs(x)=w315:dbl)
          n147 = Absolute Value(x=w317) -> (abs(x)=w318:dbl)
          n148 = Absolute Value(x=w320) -> (abs(x)=w321:dbl)
          n149 = Natural Logarithm(1:w315) -> (0:w316:dbl)
          n150 = Natural Logarithm(1:w318) -> (0:w319:dbl)
          n151 = Natural Logarithm(1:w321) -> (0:w322:dbl)
        }
        n152 = Bundle(w301, w304) -> (w298:cluster{dbl[], dbl[]})  [unwired: 1 in]
        n153 = Bundle(w301, w302) -> (w299:cluster{dbl[], dbl[]})  [unwired: 1 in]
        n154 = Bundle(w301, w303) -> (w300:cluster{dbl[], dbl[]})  [unwired: 1 in]
        n155 = call <vilib>:"Add State(s) to Queue__jki_lib_state_machine.vi"("State(s) in (\"\")"=w311) -> ("States Out"=w310:string)  [unwired: 14 in]
        n156 = Build Array(w298, w299, w300) -> (w295:cluster{dbl[], dbl[]}[])
        n157 = Bundle By Name(cluster=w296, "Arrhenius"=w295) -> (w297:T4)
      }
    }
  }
  "error out" <- w1
